vi "jMsg_SnakeProcessor_StartGame - Rx Read.vi"(8 "error in (no error)":errorcluster, 11 "jModule":refnum<class "jModule.lvclass">) -> (0 "error out":errorcluster, 3 "jModule":refnum<class "jModule.lvclass">, 7 "jMsg_SnakeProcessor_StartGame":refnum<class "jMsg_SnakeProcessor_StartGame.lvclass">)   [LabVIEW 2019, in "jMsg_SnakeProcessor_StartGame.lvclass"]
doc: "This VI is used to read data from the jMsg\n\n\nJSMA Message Wizard 0.2.0.5\nRob Humfeld - Jet Engineering\nCopyright (c) 2020, Jet Engineering"
uses:
  jMsg_SnakeProcessor_StartGame.lvclass
  <userlib>/Jet Engineering/JSMA/Libraries/jModule Class/jModule.lvclass
  <userlib>/Jet Engineering/JSMA/Libraries/jModule Class/jModule.lvclass/jModule.ctl
panel:
  in  "jMsg_SnakeProcessor_StartGame":refnum<class "jMsg_SnakeProcessor_StartGame.lvclass">
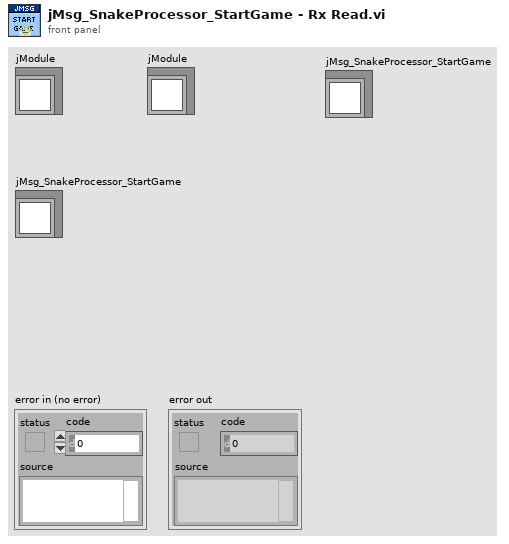
[diagram p1: front panel]
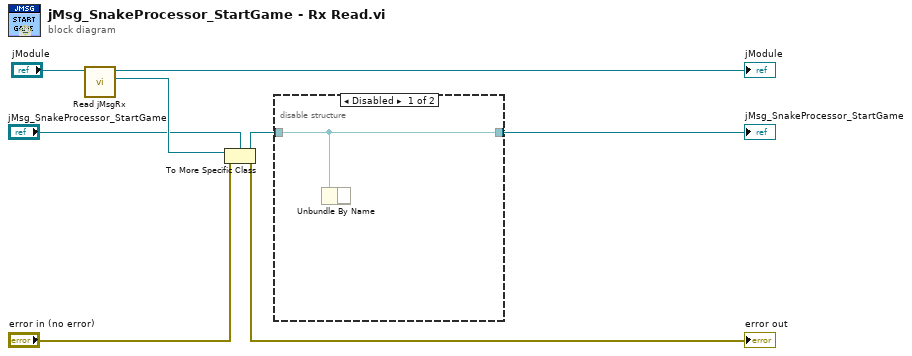
[diagram p0: block diagram]
diagram:
  n1 = call <userlib>:"Read jMsgRx.vi"("jModule in"="jModule") -> ("Received jMsg"=w5:refnum<class "jMsg.lvclass">, "jModule out"=→"jModule":refnum<class "jModule.lvclass">)  [unwired: 8 in, 1 out]
  n2 = To More Specific Class(target class="jMsg_SnakeProcessor_StartGame", reference=w5, error in="error in (no error)") -> (specific class reference=w3:refnum<class "jMsg_SnakeProcessor_StartGame.lvclass">, error out=→"error out":errorcluster)
  n3 = disable-structure shown="Disabled" {
    disable-tunnel: w3 -> [w9 w10]
    disable-tunnel: [w9 w10] -> w8
    frame Disabled {
      n4 = Unbundle By Name(w9) -> ()  [unwired: 1 out]
    }
    frame Enabled {
    }
  }
  "jMsg_SnakeProcessor_StartGame" <- w8
